vi "Set Default.vi"(8 "error in (no error)":errorcluster, 11 "DMM Config Trigger Msg in":refnum<class "DMM Config Trigger Msg.lvclass">) -> (0 "error out":errorcluster, 3 "DMM Config Trigger Msg out":refnum<class "DMM Config Trigger Msg.lvclass">)   [LabVIEW 2020, in "DMM Msg.lvlib" / "DMM Config Trigger Msg.lvclass"]
doc: "Restore private data to a defined default state.\n\nThis implementation sets:\nTriggers to measure and Samples per Trigger 1\nTrigger Type Index 0\nSample Interval -1\nAwait reply, -1ms timeout at normal priority without publish"
uses:
  DMM Config Trigger Msg.lvclass
  PPL/HDH.Actor Framework.Core.Actor.lvlibp/1abvi3w/vi.lib/ActorFramework/Message Enqueuer/Message Priority.ctl
  PPL/HDH.Actor Framework.Core.Publisher.lvlibp/Messages/Response Msg/Response Core/Controls/Ctl_SendFunction.ctl
  DMM Config Trigger Msg.lvclass/DMM Config Trigger Msg.ctl
  DMM Msg/DMM Msg.lvclass
  PPL/HDH.Actor Framework.Core.Instrument Handler.lvlibp/Messages/Instrument Msg/Instrument Msg.lvclass
  PPL/HDH.Actor Framework.Core.Publisher.lvlibp
  PPL/HDH.Actor Framework.Core.Actor.lvlibp/1abvi3w/vi.lib/ActorFramework/Message Enqueuer/Message Enqueuer.lvclass
  C:/Current projects/WS/PPL/HDH.Actor Framework.Core.Instrument Handler.lvlibp/Messages/Instrument Msg/Instrument Msg.lvclass
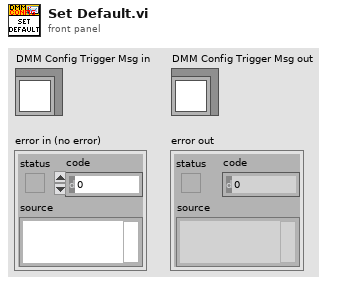
[diagram p1: front panel]
types:
  T1 = typedef "HDH.Actor Framework.Core.Publisher.lvlibp/Ctl_SendFunction.ctl" = enum16{"Send and Forget", "Request Reply", "Await Reply"}
  T2 = typedef "HDH.Actor Framework.Core.Actor.lvlibp/Message Enqueuer.lvclass/Message Priority.ctl" = enum16{"Low", "Normal", "High"}
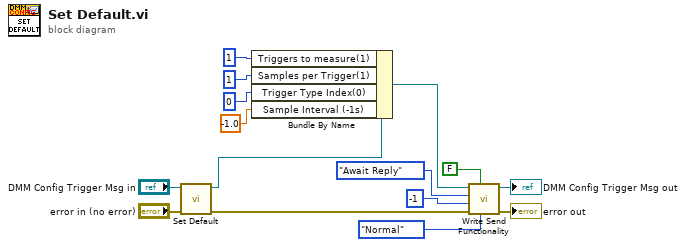
[diagram p0: block diagram]
diagram:
  n1 = call-parent "Set Default.vi"("error in (no error)"="error in (no error)", "Flex Msg in"="DMM Config Trigger Msg in") -> ("error out"=w9:errorcluster, "Flex Msg out"=w15:refnum<class "DMM Config Trigger Msg.lvclass">)  [unwired: 8 in]
  n2 = Bundle By Name(cluster=w15, "Triggers to measure(1)"=1, "Samples per Trigger(1)"=1, "Trigger Type Index(0)"=u16 0, "Sample Interval (-1s)"=-1.0) -> (w12:refnum<class "DMM Config Trigger Msg.lvclass">)
  n3 = call "Write Send Functionality.vi"("Message Priority(Normal)"=Message_Priority."Normal", "Publish Data?(T)"=FALSE, "error in (no error)"=w9, "Timeout if Waiting(-1ms)"=-1, "Send Function(Await Reply)"=Ctl_SendFunction."Await Reply", "Instrument Msg in"=w12) -> ("error out"=→"error out":errorcluster, "Instrument Msg out"=→"DMM Config Trigger Msg out":refnum<class "DMM Config Trigger Msg.lvclass">)  [unwired: 4 in]
